vi "OldMotorTEST.vi"() -> ()   [LabVIEW 2019]
uses:
  KNRm_ReMi_OS5.lvlibp/KNRm_ReMi_Toolkit/IO/LowLevel/IO_Channel_Motor.ctl
  KNRm_ReMi_OS5.lvlibp
panel:
  out "ENC (deg)":dbl
  in  "stop":bool
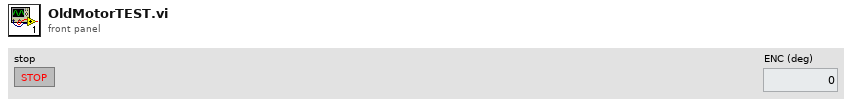
[diagram p1: front panel]
types:
  T1 = typedef "KNRm_ReMi_OS5.lvlibp/IO_Channel_Motor.ctl" = enum16{"M1", "M2", "M3", "M4"}
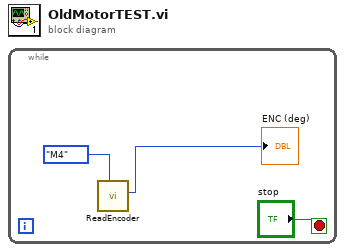
[diagram p0: block diagram]
diagram:
  n1 = while {
    stop <- "stop" stop-if-true
    n2 = call "ReadEncoder.vi"("Channel"=IO_Channel_Motor."M4") -> ("ENC (count)"=→"ENC (deg)":i32)  [unwired: 9 in, 1 out]
  }
